vi "Read handle.vi"(8 "error in (no error)":errorcluster, 11 "Synnax Client in":refnum<class "Synnax Client.lvclass">) -> (0 "error out":errorcluster, 2 "handle":u64, 3 "Synnax Client out":refnum<class "Synnax Client.lvclass">)   [LabVIEW 2026, in "synnax_lib.lvlib" / "Synnax Client.lvclass"]
uses:
  Synnax Client.lvclass
  Synnax Client.lvclass/Synnax Client.ctl
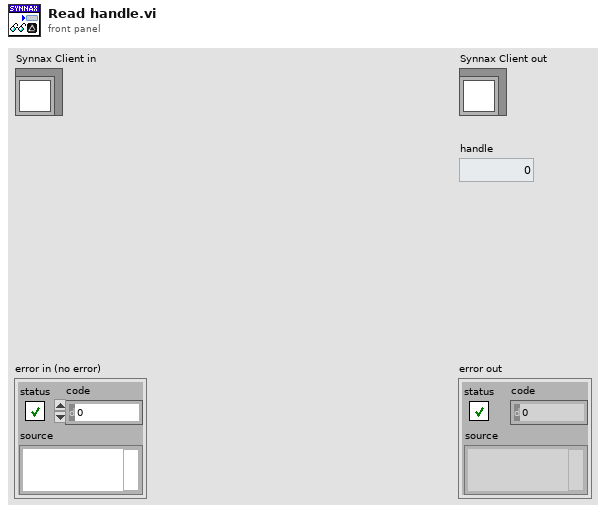
[diagram p1: front panel]
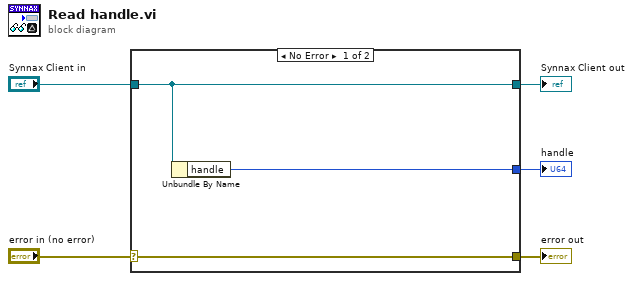
[diagram p0: block diagram]
diagram:
  n1 = case shown="No Error" "error in (no error)" {
    selector: "error in (no error)" -> [w8 w9]
    tunnel: [w8 w9] -> w4
    tunnel: [w7 w10] -> w2
    tunnel: "Synnax Client in" -> [w7 w10]
    tunnel: [w6 _] -> w1
    frame No Error {
      n2 = Unbundle By Name(w7) -> ("handle"=w6:u64)
    }
    frame Error {
    }
  }
  "error out" <- w4
  "Synnax Client out" <- w2
  "handle" <- w1
